vi "SaveForPreviousVersion.vi"() -> ()   [LabVIEW 2018]
panel:
  out "Success":bool=TRUE
  in  "Version":string(combo)="16.0"
  in  "Destination Path":path=path "D:/HardwareRevamp/Test"
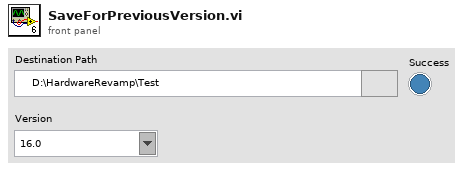
[diagram p1: front panel]
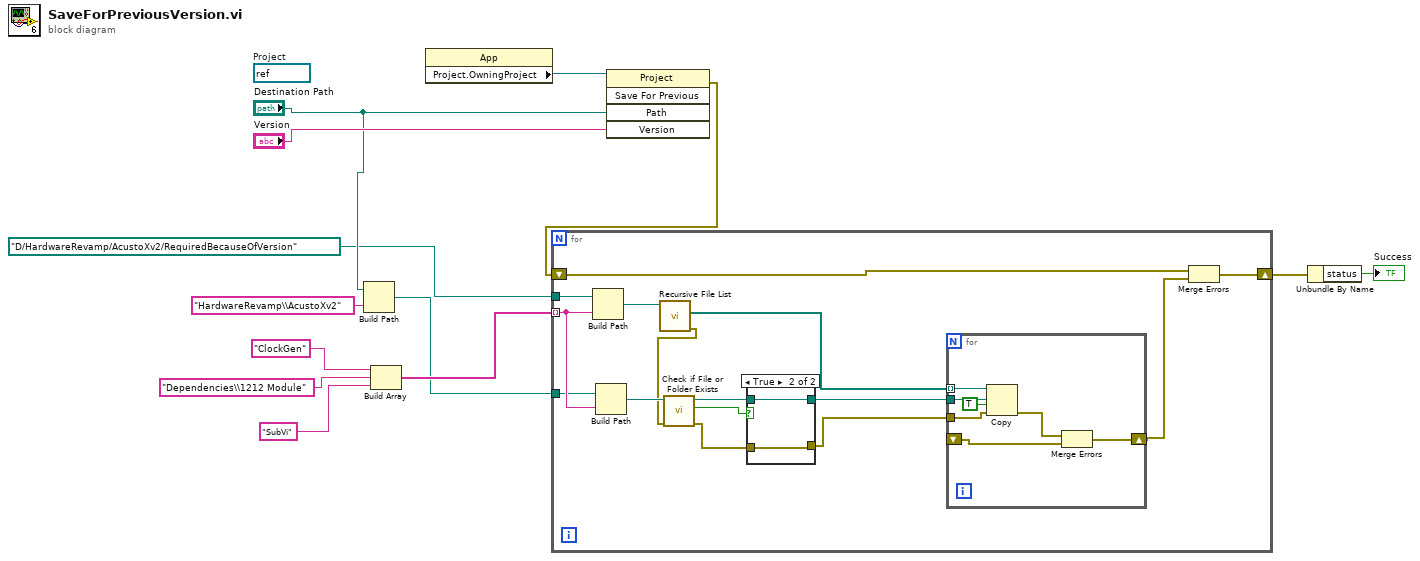
[diagram p0: block diagram]
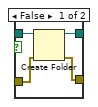
[diagram p2: hidden frame]
diagram:
  (unwired) refnum<vi> refnum  # Project
  n1 = Build Path(base path="Destination Path", name or relative path="HardwareRevamp\\AcustoXv2") -> (appended path=w6:path)
  n2 = Build Array("ClockGen" ("name or relative path"), "Dependencies\\1212 Module" ("name or relative path"), "SubVi" ("element")) -> (w7:string[])
  n3 = property class="App"() -> ("Project.OwningProject"=w5:refnum<vi>)  [unwired: 2 in, 2 out]
  n4 = invoke class="Project" method="Save For Previous"(reference=w5, "Path"="Destination Path", "Version"="Version") -> (error out=w3:errorcluster)  [unwired: 2 in, 4 out]
  n5 = for {
    tunnel: path "D:/HardwareRevamp/AcustoXv2/RequiredBecauseOfVersion" ("Source Folder") -> [w28]
    tunnel: w7 -> [w27] mode=indexing
    tunnel: w6 -> [w22]
    shift-right: [w15] -> w2
    shift-left: w3 -> [w14]
    n6 = Build Path(base path=w28, name or relative path=w27) -> (appended path=w25:path)
    n7 = Build Path(base path=w22, name or relative path=w27) -> (appended path=w21:path)
    n8 = call <vilib>:"Recursive File List.vi"("Folder Path"=w25) -> ("error out"=w17:errorcluster, "All Files in Dir"=w26:path[])  [unwired: 6 in, 3 out]
    n9 = call <vilib>:"Check if File or Folder Exists.vi"("error in (no error)"=w17, "path"=w21) -> ("error out"=w19:errorcluster, "file or folder exists?"=w23:bool, "dup path"=w24:path)  [unwired: 7 in]
    n10 = case shown="True" w23 {
      tunnel: w24 -> [w32 w34]
      tunnel: [w31 w34] -> w20
      tunnel: w19 -> [w30 w33]
      tunnel: [w29 w33] -> w18
      frame False {
        n11 = Create Folder(path (use dialog)=w32, error in=w30) -> (created path=w31:path, error out=w29:errorcluster)  [unwired: 1 in, 1 out]
      }
      frame True {
      }
    }
    n12 = for {
      tunnel: w26 -> [w41] mode=indexing
      tunnel: w20 -> [w39]
      tunnel: w18 -> [w38]
      shift-right: [w36] -> w16
      shift-left: _ -> [w35]
      n13 = Copy(8:w38, 9:TRUE ("overwrite (F)"), 10:w39, 11:w41) -> (0:w37:errorcluster)  [unwired: 1 in, 2 out]
      n14 = Merge Errors(w37, w35) -> (w36:errorcluster)
    }
    n15 = Merge Errors(w14, w16) -> (w15:errorcluster)
  }
  n16 = Unbundle By Name(w2) -> ("status"=→"Success":bool)
